vi "Frequency.vi"() -> ()   [LabVIEW 2016]
uses:
  <vilib>/measure/matone.llb/Extract Single Tone Information N Chan.vi
  <vilib>/measure/NI_MABase.lvlib
  <vilib>/measure/NI_MAPro.lvlib
panel:
  out "detected frequencies":dbl[](array[numeric]) format="%.2p"
  out "detected amplitudes":dbl[](array[numeric]) format="%.2p"
  out "detected phases (deg)":dbl[](array[numeric]) format="%.2p"
  in  "signal type":T1(ring)
  out "data 2":dynamicdata(graph) caption="data"
  out "data":dynamicdata(graph)
  in  "sampling info":cluster{"Fs":dbl, "#s":dbl}={"Fs"=1000.0, "#s"=1000.0} {"Fs" format="%.2p"}
  in  "stop":bool
  in  "phase":dbl format="%.2p"
  in  "amplitude":dbl=1.0 format="%0.2p"
  in  "frequency":dbl=10.0 format="%0.2p"
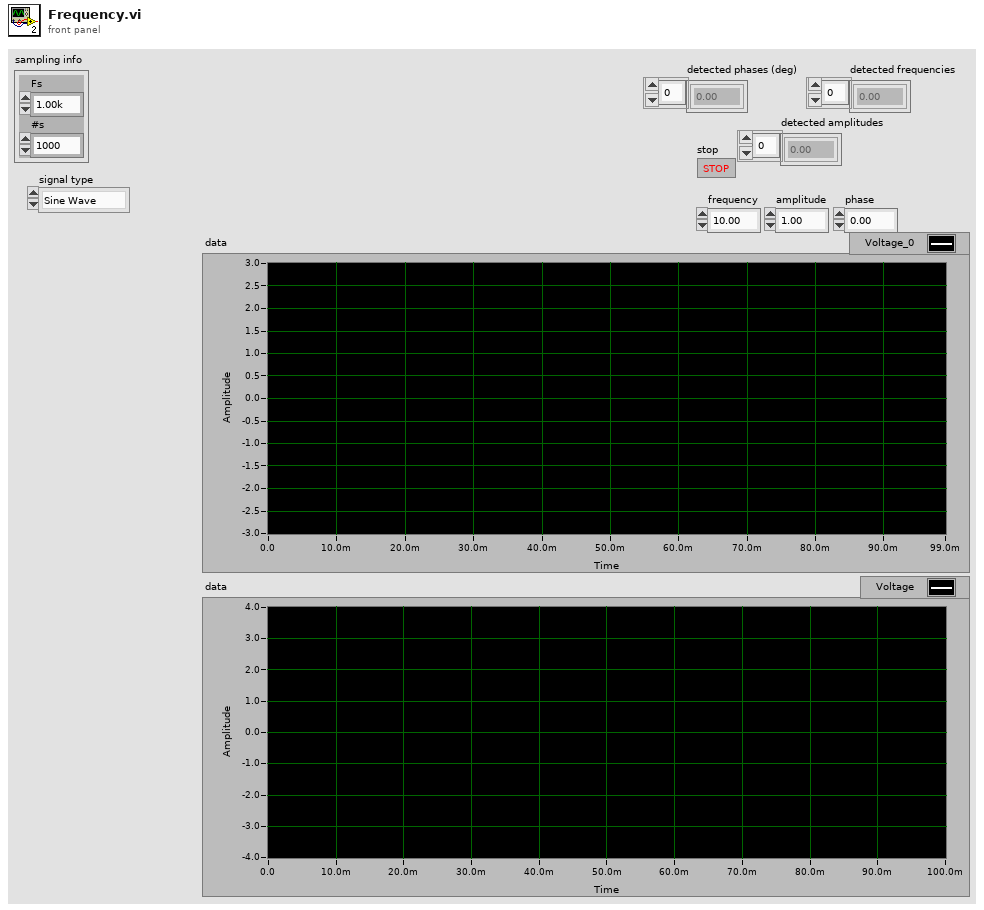
[diagram p1: front panel]
types:
  T1 = enum16{"Sine Wave", "Triangle Wave", "Square Wave", "Sawtooth Wave"}
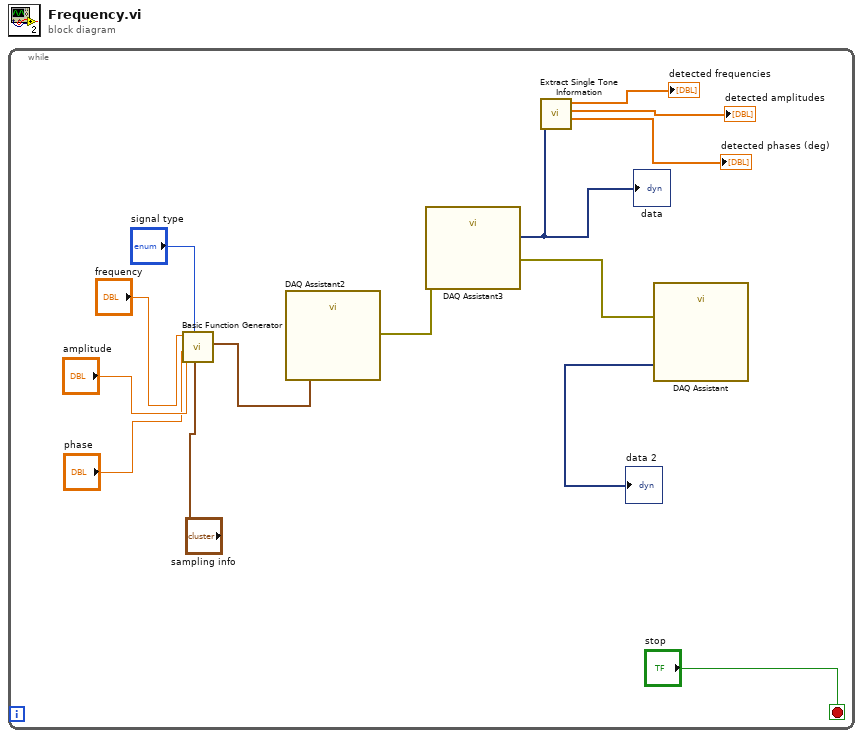
[diagram p0: block diagram]
diagram:
  n1 = while {
    stop <- "stop" stop-if-true
    n2 = call <vilib>:"Basic Function Generator.vi"("sampling info"="sampling info", "signal type"="signal type", "phase"="phase", "amplitude"="amplitude", "frequency"="frequency") -> ("signal out"=w9:waveform(dbl))  [unwired: 4 in, 2 out]
    n3 = call "DAQ Assistant2"("data"=w9) -> ("error out"=w13:errorcluster)  [unwired: 16 in, 2 out]
    n4 = call "DAQ Assistant3"("error in"=w13) -> ("data"=w4:dynamicdata, "error out"=w11:errorcluster)  [unwired: 16 in, 1 out]
    "data" <- w4
    n5 = call-poly <vilib>:"Extract Single Tone Information.vi"("time signals in"=w4) -> ("detected phases (deg)"=→"detected phases (deg)":dbl[], "detected amplitudes"=→"detected amplitudes":dbl[], "detected frequencies"=→"detected frequencies":dbl[])  [unwired: 5 in, 3 out]
    n6 = call "DAQ Assistant"("error in"=w11) -> ("data"=→"data 2":dynamicdata)  [unwired: 16 in, 2 out]
  }
